vi "zi-read.vi"(8 "error in (no error)":errorcluster, 11 "ZI Lockin in":refnum<class "ZI Lockin.lvclass">) -> (0 "error out":errorcluster, 2 "Result":dbl, 3 "ZI Lockin out":refnum<class "ZI Lockin.lvclass">)   [LabVIEW 2016, in "ZI Lockin.lvclass"]
uses:
  ZI Lockin.lvclass
  Read ZI Handle.vi
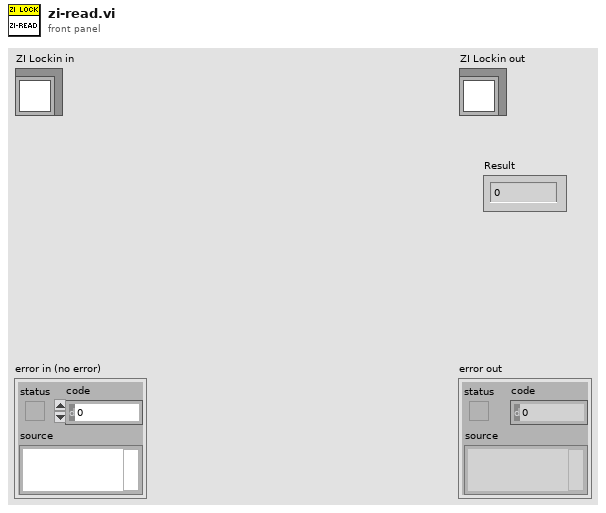
[diagram p1: front panel]
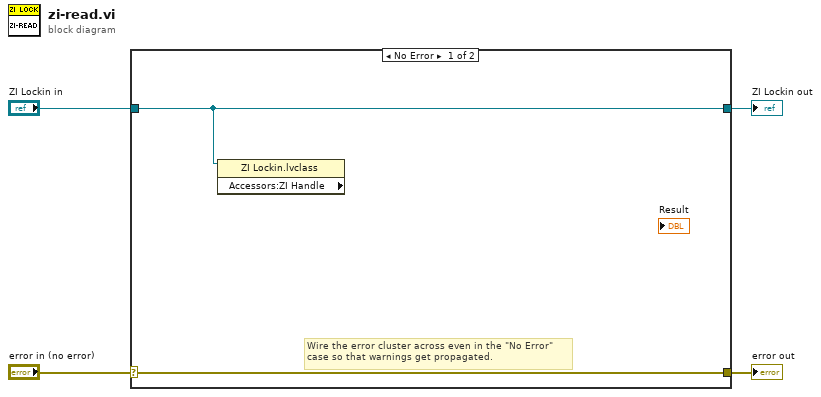
[diagram p0: block diagram]
diagram:
  n1 = case shown="No Error" "error in (no error)" {
    selector: "error in (no error)" -> [w6 w8]
    tunnel: [w6 w8] -> w3
    tunnel: [w5 w7] -> w1
    tunnel: "ZI Lockin in" -> [w5 w7]
    frame No Error {
      # "Wire the error cluster across even in the \"No Error\"\ncase so that warnings get propagated."
      n2 = property class="ZI Lockin.lvclass" props=["Accessors:ZI Handle"](reference=w5) -> ()  [unwired: 1 in, 3 out]
    }
    frame Error {
    }
  }
  "error out" <- w3
  "ZI Lockin out" <- w1
